vi "Demo - Shortcuts - Pt2.vi"() -> ()   [LabVIEW 2020]
panel:
  out "Create Space":dbl
  in  "VISA in":refnum<visa-resource-name>
  # "LabVIEW Shortcuts - Pt2"
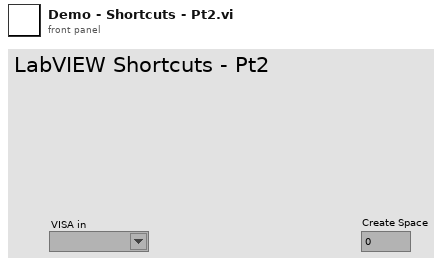
[diagram p1: front panel]
types:
  T1 = enum16{"Coding - Copy Code", "Coding - Create Space in Diagram", "Coding - Expand Contract Structures", "Coding - Distribute Code", "Coding - Align items", "Coding - Move Items", "Coding - Tool Selection Color Grab", "Coding - Text Increase decrease font", "Coding - Open SubVI FP and BD", "Coding - Find something, next or prev", "Coding - Error Window List", "Coding - Show all windows", "Coding - Class Browser"}
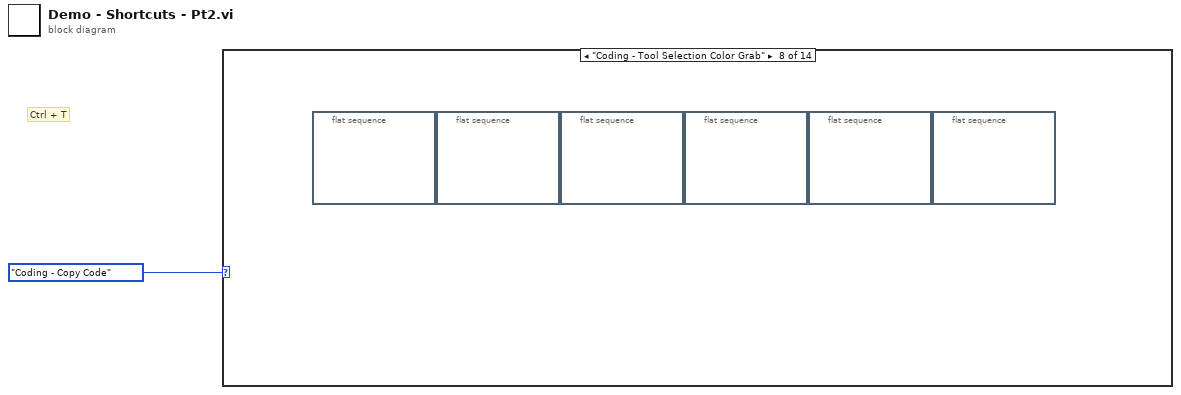
[diagram p0: block diagram]
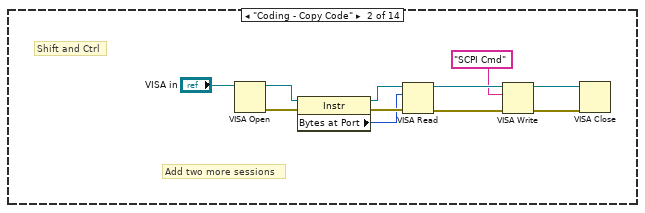
[diagram p3: hidden frame]
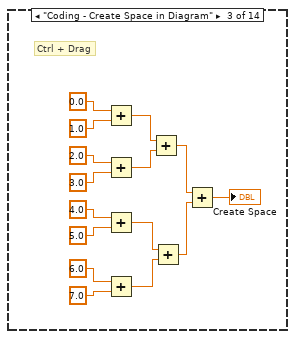
[diagram p4: hidden frame]
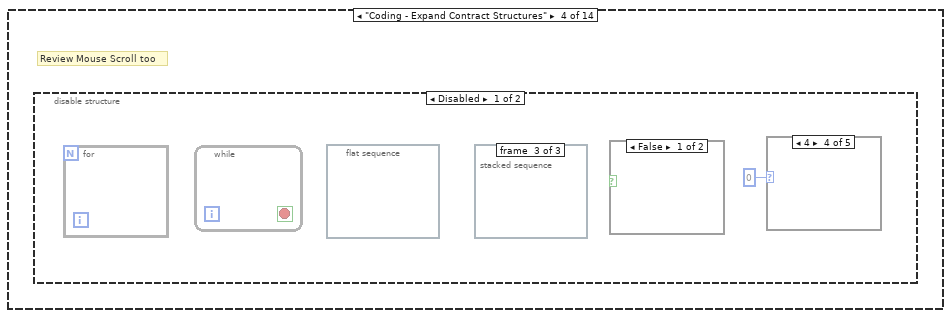
[diagram p5: hidden frame]
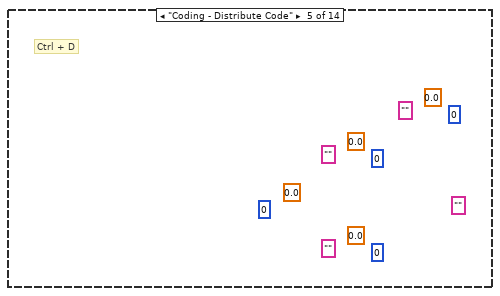
[diagram p14: hidden frame]
diagram:
  # "Ctrl + T"
  n1 = case shown="\"Coding - Tool Selection Color Grab\"" T1."Coding - Copy Code" {
    frame Default {
    }
    frame "Coding - Copy Code" {
      # "Shift and Ctrl"
      # "Add two more sessions"
      n2 = VISA Open(VISA resource name="VISA in") -> (VISA resource name=w8:refnum<visa-resource-name>, error out=w11:errorcluster)  [unwired: 4 in]
      n3 = property class="Instr"(reference=w8, error in=w11) -> (reference out=w7:refnum<visa-resource-name>, error out=w9:errorcluster, "Bytes at Port"=w6:u32)
      n4 = VISA Read(VISA resource name=w7, byte count=w6, error in (no error)=w9) -> (VISA resource name out=w4:refnum<visa-resource-name>, error out=w10:errorcluster)  [unwired: 2 out]
      n5 = VISA Write(VISA resource name=w4, write buffer="SCPI Cmd", error in (no error)=w10) -> (VISA resource name out=w3:refnum<visa-resource-name>, error out=w5:errorcluster)  [unwired: 1 out]
      n6 = VISA Close(VISA resource name=w3, error in (no error)=w5) -> ()  [unwired: 1 out]
    }
    frame "Coding - Create Space in Diagram" {
      # "Ctrl + Drag"
      n7 = Add(x=0.0, y=1.0) -> (x+y=w16:dbl)
      n8 = Add(x=2.0, y=3.0) -> (x+y=w17:dbl)
      n9 = Add(x=4.0, y=5.0) -> (x+y=w19:dbl)
      n10 = Add(x=6.0, y=7.0) -> (x+y=w18:dbl)
      n11 = Add(x=w16, y=w17) -> (x+y=w15:dbl)
      n12 = Add(x=w19, y=w18) -> (x+y=w14:dbl)
      n13 = Add(x=w15, y=w14) -> (x+y=→"Create Space":dbl)
    }
    frame "Coding - Expand Contract Structures" {
      # "Review Mouse Scroll too"
      n14 = disable-structure shown="Disabled" {
        frame Disabled {
          n15 = for {
          }
          n16 = while {
            stop <- _ stop-if-true
          }
          n17 = flat-sequence {
            frame #0 {
            }
          }
          n18 = stacked-sequence {
            frame #0 {
            }
            frame #1 {
            }
            frame #2 {
            }
          }
          n19 = case shown="False" {
            selector: _ -> [_ _]
            frame False {
            }
            frame True {
            }
          }
          n20 = case shown="4" 0 {
            frame 0, Default {
            }
            frame 2 {
            }
            frame 3 {
            }
            frame 4 {
            }
            frame 1 {
            }
          }
        }
        frame Enabled {
        }
      }
    }
    frame "Coding - Distribute Code" {
      (unwired) 0.0
      (unwired) ""
      (unwired) 0
      (unwired) 0.0
      (unwired) ""
      (unwired) 0
      (unwired) 0.0
      (unwired) ""
      (unwired) 0
      (unwired) 0.0
      (unwired) ""
      (unwired) 0
      # "Ctrl + D"
    }
    frame "Coding - Align items" {
      # "Ctrl + Shift + A"
    }
    frame "Coding - Move Items" {
      # "Direction Keys\nDirection Keys + Shift"
    }
    frame "Coding - Tool Selection Color Grab" {
      n21 = flat-sequence {
        frame #0 {
        }
      }
      n22 = flat-sequence {
        frame #0 {
        }
      }
      n23 = flat-sequence {
        frame #0 {
        }
      }
      n24 = flat-sequence {
        frame #0 {
        }
      }
      n25 = flat-sequence {
        frame #0 {
        }
      }
      n26 = flat-sequence {
        frame #0 {
        }
      }
    }
    frame "Coding - Text Increase decrease font" {
    }
    frame "Coding - Open SubVI FP and BD" {
    }
    frame "Coding - Find something, next or prev" {
    }
    frame "Coding - Error Window List" {
    }
    frame "Coding - Show all windows" {
    }
    frame "Coding - Class Browser" {
    }
  }
